vi "RSZVB Set User Defined Preset State.vi"(8 "error in (no error)":errorcluster {"code" format="%.0x"}, 10 "User Defined Preset (F: Off)":bool, 11 "VISA session":refnum<visa-resource-name>) -> (0 "error out":errorcluster {"code" format="%.0x"}, 3 "dup VISA session":refnum<visa-resource-name>)   [LabVIEW 2011]
doc: "This VI selects a factory preset or a user-defined preset.\n\nRemote-control command(s):\nSYSTem:PRESet:USER[:STATe] ON | OFF"
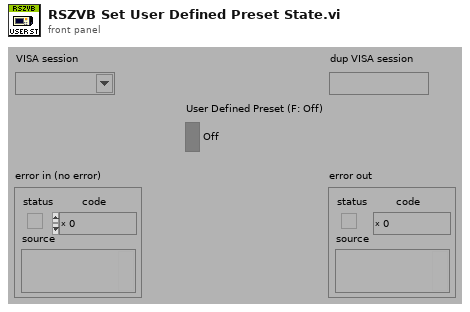
[diagram p1: front panel]
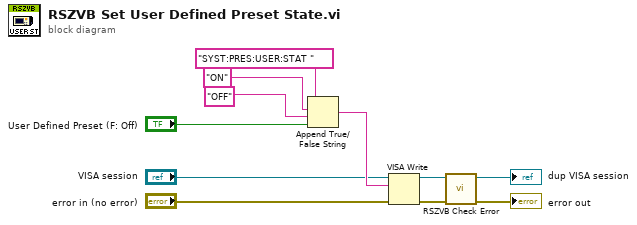
[diagram p0: block diagram]
diagram:
  n1 = Append True/False String(1:"User Defined Preset (F: Off)", 2:"OFF", 3:"ON", 4:"SYST:PRES:USER:STAT ") -> (0:w6:string)
  n2 = VISA Write(VISA resource name="VISA session", write buffer=w6, error in (no error)="error in (no error)") -> (VISA resource name out=w10:refnum<visa-resource-name>, error out=w11:errorcluster)  [unwired: 1 out]
  n3 = call "RSZVB Check Error.vi"("error in (no error)"=w11, "VISA session"=w10) -> ("error out"=→"error out":errorcluster, "dup VISA session"=→"dup VISA session":refnum<visa-resource-name>)  [unwired: 8 in]
